vi "DataSave.vi"(0 "DeviceNo":u32, 1 "FileName":string, 2 "Slide Refnum":refnum<vi>, 5 "ChildNo":u32, 9 "Rate":i32=30, 11 "error in (no error)":errorcluster, 12 "ShowCompreddDlg":u32, 13 "File_Frame":cluster{"StartFrame":i32, "EndFrame":i32}) -> (6 "Cancel?":bool, 8 "Error?":bool, 15 "Error_Out":T1)   [LabVIEW 2015]
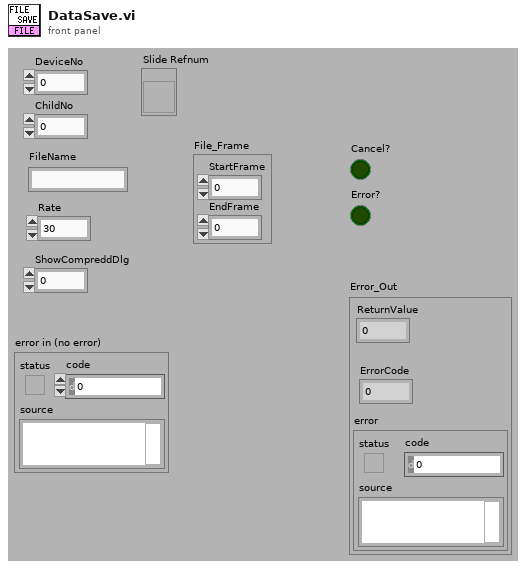
[diagram p1: front panel]
types:
  T1 = cluster{"ReturnValue":u32, "ErrorCode":u32, "error ":errorcluster}
  T2 = cluster{"return type":u32, "pErrorCode":u32, "error ":errorcluster}
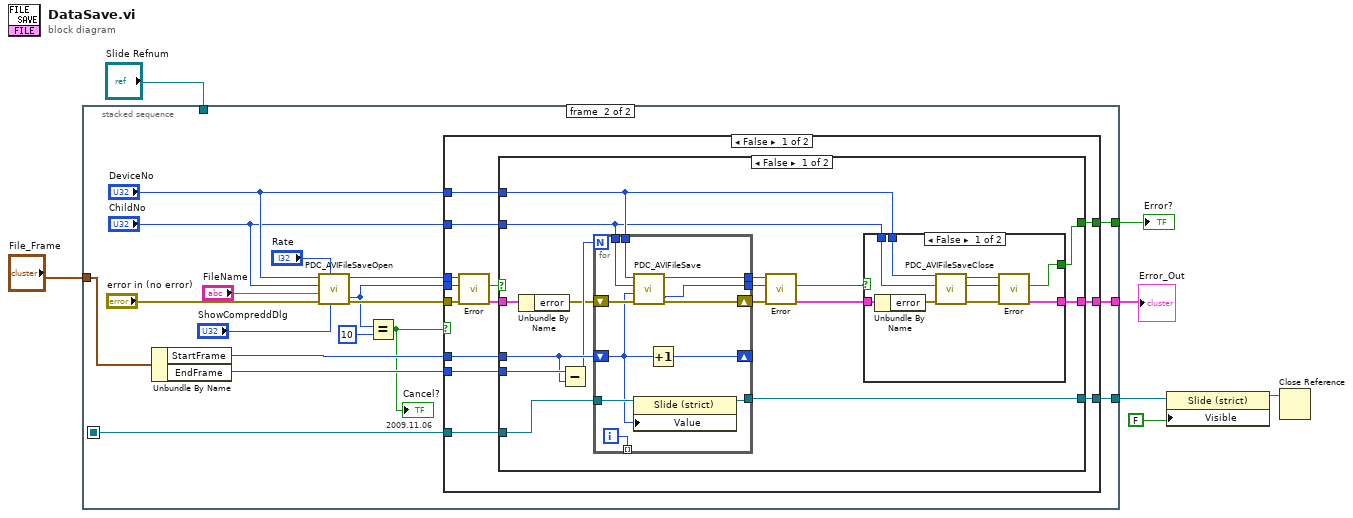
[diagram p0: block diagram]
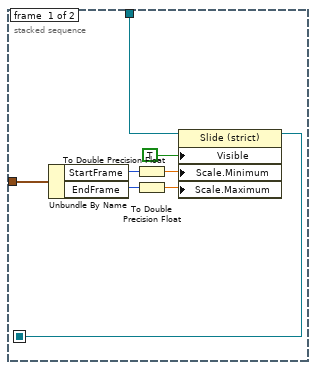
[diagram p2: hidden frame]
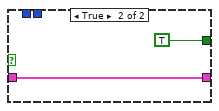
[diagram p3: hidden frame]
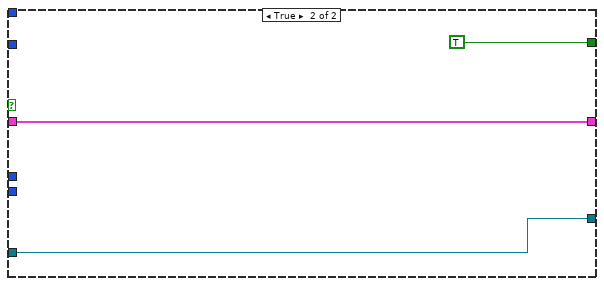
[diagram p4: hidden frame]
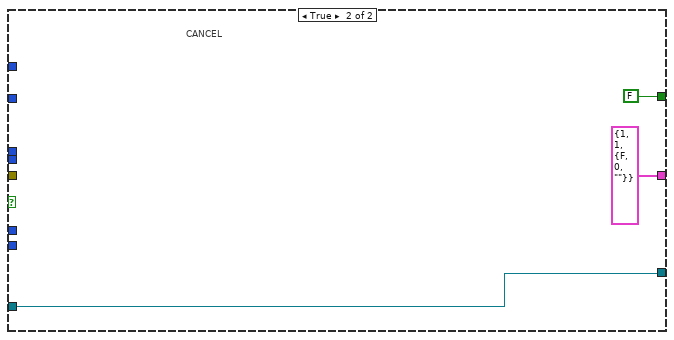
[diagram p5: hidden frame]
diagram:
  n1 = stacked-sequence {
    seq-local: [w13 _] -> [_ w28]
    tunnel: "Slide Refnum" -> [w15 _]
    tunnel: "File_Frame" -> [w12 w26]
    tunnel: [_ w21] -> w6
    tunnel: [_ w20] -> w5
    tunnel: [_ w19] -> w2
    frame #0 {
      n2 = Unbundle By Name(w12) -> ("StartFrame"=w11:i32, "EndFrame"=w10:i32)
      n3 = To Double Precision Float(number=w11) -> (double precision float=w9:dbl)
      n4 = To Double Precision Float(number=w10) -> (double precision float=w8:dbl)
      n5 = property class="Slide (strict)"(reference=w15, "Visible"=TRUE ("表示"), "Scale.Minimum"=w9, "Scale.Maximum"=w8) -> (reference out=w13:refnum<vi>)  [unwired: 1 in, 1 out]
    }
    frame #1 {
      # "2009.11.06"
      n6 = Unbundle By Name(w26) -> ("StartFrame"=w24:i32, "EndFrame"=w25:i32)
      n7 = call "PDC_AVIFileSaveOpen.vi"("ShowCompressDlg"="ShowCompreddDlg", "Rate"="Rate", "error in (no error)"="error in (no error)", "FileName"="FileName", "ChildNo"="ChildNo", "DeviceNo"="DeviceNo") -> ("error out"=w23:errorcluster, "ReturnValue"=w22:u32, "ErrorCode"=w18:u32)  [unwired: 3 out]
      n8 = Equal?(x=w18, y=u32 10) -> (x = y?=w16:bool)
      "Cancel?" <- w16
      n9 = case shown="False" w16 {
        tunnel: "DeviceNo" -> [w46 _]
        tunnel: "ChildNo" -> [w45 _]
        tunnel: w28 -> [w44 w88]
        tunnel: w25 -> [w43 _]
        tunnel: w24 -> [w42 _]
        tunnel: w23 -> [w41 _]
        tunnel: w22 -> [w40 _]
        tunnel: [w37 T2 {"return type"=1, "pErrorCode"=1, "error "={"status"=FALSE, "code"=0, "source"=""}} ("Error_Out")] -> w21
        tunnel: [w36 FALSE ("Error?")] -> w20
        tunnel: [w35 w88] -> w19
        tunnel: w18 -> [w34 _]
        frame False {
          n10 = call "Error.vi"("error in (no error)"=w41, "ErrorCode"=w34, "ReturnValue"=w40) -> ("Error_Out"=w38:T1, "Error?"=w39:bool)  [unwired: 7 out]
          n11 = case shown="False" w39 {
            tunnel: w46 -> [w62 _]
            tunnel: w45 -> [w61 _]
            tunnel: w44 -> [w60 w85]
            tunnel: w43 -> [w59 _]
            tunnel: w42 -> [w58 _]
            tunnel: w38 -> [w56 w87]
            tunnel: [w47 w87] -> w37
            tunnel: [w49 TRUE] -> w36
            tunnel: [w54 w85] -> w35
            frame False {
              n12 = Unbundle By Name(w56) -> ("error"=w55:errorcluster)
              n13 = Subtract(x=w59, y=w58) -> (x-y=w57:i32)
              n14 = for {
                N: w57 -> [_]
                tunnel: w62 -> [w82]
                tunnel: w61 -> [w81]
                shift-right: [w80] -> _
                shift-left: w58 -> [w78]
                tunnel: w60 -> [w79]
                tunnel: [w77] -> w54
                tunnel: [w76] -> _ mode=indexing
                shift-right: [w83] -> w51
                shift-left: w55 -> [w84]
                tunnel: [w75] -> w53
                tunnel: [w74] -> w52
                i -> [w76]
                n15 = call "PDC_AVIFileSave.vi"("error in (no error)"=w84, "FrameNo"=w78, "ChildNo"=w81, "DeviceNo"=w82) -> ("error out"=w83:errorcluster, "ReturnValue"=w75:u32, "ErrorCode"=w74:u32)  [unwired: 5 out]
                n16 = property class="Slide (strict)"(reference=w79, "Value"=w78) -> (reference out=w77:refnum<vi>)  [unwired: 1 in, 1 out]
                n17 = Increment(x=w78) -> (x+1=w80:i32)
              }
              n18 = call "Error.vi"("error in (no error)"=w51, "ErrorCode"=w52, "ReturnValue"=w53) -> ("Error_Out"=w48:T1, "Error?"=w50:bool)  [unwired: 7 out]
              n19 = case shown="False" w50 {
                tunnel: w62 -> [w71 _]
                tunnel: w61 -> [w70 _]
                tunnel: [w63 TRUE] -> w49
                tunnel: w48 -> [w69 w72]
                tunnel: [w64 w72] -> w47
                frame False {
                  n20 = Unbundle By Name(w69) -> ("error"=w68:errorcluster)
                  n21 = call "PDC_AVIFileSaveClose.vi"("error in (no error)"=w68, "ChildNo"=w70, "DeviceNo"=w71) -> ("error out"=w65:errorcluster, "ReturnValue"=w67:u32, "ErrorCode"=w66:u32)  [unwired: 6 out]
                  n22 = call "Error.vi"("error in (no error)"=w65, "ErrorCode"=w66, "ReturnValue"=w67) -> ("Error_Out"=w64:T1, "Error?"=w63:bool)  [unwired: 7 out]
                }
                frame True {
                }
              }
            }
            frame True {
            }
          }
        }
        frame True {
          # "CANCEL"
        }
      }
    }
  }
  "Error_Out" <- w6
  "Error?" <- w5
  n23 = property class="Slide (strict)"(reference=w2, "Visible"=FALSE ("表示")) -> (reference out=w4:refnum<vi>)  [unwired: 1 in, 1 out]
  n24 = Close Reference(reference=w4) -> ()  [unwired: 1 in, 1 out]
